vi "CRYSet Graph Data in Graph.vi"(10 "pGraph VI":refnum<vi>, 11 "Flatten Data String":string) -> ()   [LabVIEW 2013]
uses:
  Control/CRYPicture Property.ctl
panel:
  in  "Picture Property":T1
  in  "Text Format":T2
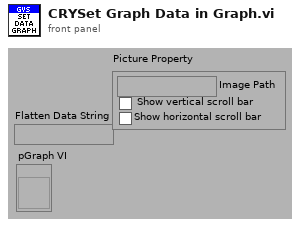
[diagram p1: front panel]
types:
  T1 = typedef "CRYPicture Property.ctl" = cluster{"Image Path":string, "Show vertical scroll bar":bool, "Show horizontal scroll bar":bool}
  T2 = cluster{"Size":u32, "Bold":bool, "Italic":bool, "Underline":bool, "Strikethrough":bool, "Color":u32, "Font":string, "String":string}
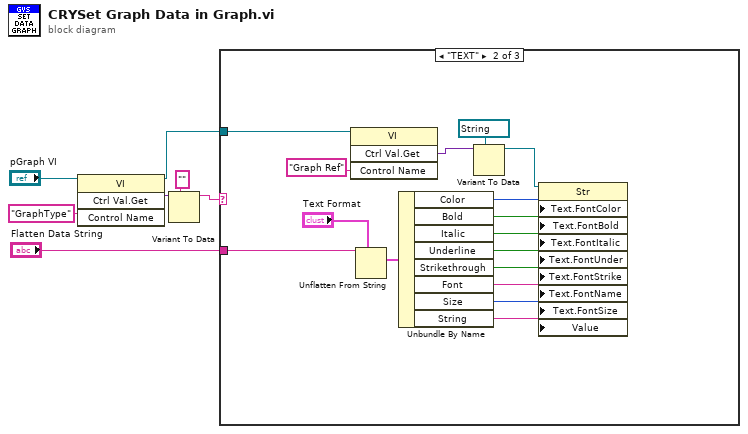
[diagram p0: block diagram]
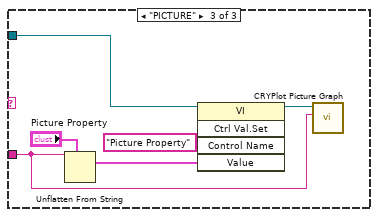
[diagram p3: hidden frame]
diagram:
  n1 = invoke class="VI" method="Ctrl Val.Get"(reference="pGraph VI", "Control Name"="GraphType") -> (reference out=w1:refnum<vi>, "Get Control Value Variant"=w6:variant)  [unwired: 2 in, 2 out]
  n2 = Variant To Data(type="", Variant=w6) -> (data=w3:string)  [unwired: 1 in, 1 out]
  n3 = case shown="\"TEXT\"" w3 {
    tunnel: "Flatten Data String" -> [_ w23 w26]
    tunnel: w1 -> [_ w11 w25]
    frame Default {
    }
    frame "TEXT" {
      n4 = invoke class="VI" method="Ctrl Val.Get"(reference=w11, "Control Name"="Graph Ref") -> ("Get Control Value Variant"=w9:variant)  [unwired: 2 in, 3 out]
      n5 = Unflatten From String(type="Text Format", binary string=w23) -> (value=w21:T2)  [unwired: 3 in, 2 out]
      n6 = Unbundle By Name(w21) -> ("Color"=w20:u32, "Bold"=w19:bool, "Italic"=w18:bool, "Underline"=w17:bool, "Strikethrough"=w16:bool, "Font"=w15:string, "Size"=w14:u32, "String"=w13:string)
      n7 = Variant To Data(type=refnum<vi> refnum ("WaveGraph Ref"), Variant=w9) -> (data=w8:refnum<vi>)  [unwired: 1 in, 1 out]
      n8 = property class="Str"(reference=w8, "Text.FontColor"=w20, "Text.FontBold"=w19, "Text.FontItalic"=w18, "Text.FontUnder"=w17, "Text.FontStrike"=w16, "Text.FontName"=w15, "Text.FontSize"=w14, "Value"=w13) -> ()  [unwired: 1 in, 2 out]
    }
    frame "PICTURE" {
      n9 = Unflatten From String(type="Picture Property", binary string=w26) -> (value=w27:T1)  [unwired: 3 in, 2 out]
      n10 = invoke class="VI" method="Ctrl Val.Set"(reference=w25, "Control Name"="Picture Property", "Value"=w27) -> (reference out=w24:refnum<vi>)  [unwired: 2 in, 4 out]
      n11 = call "CRYPlot Picture Graph.vi"("Flattened Property"=w26, "pGraph VI In"=w24) -> ()  [unwired: 10 in]
    }
  }
